vi "unflatten.vi"(8 "error in":errorcluster, 10 "flattened system":string) -> (0 "error out":errorcluster, 3 "test-system out":refnum<class "test-system.lvclass">)   [LabVIEW 2020, in "test-system.lvclass"]
uses:
  test-system.lvclass
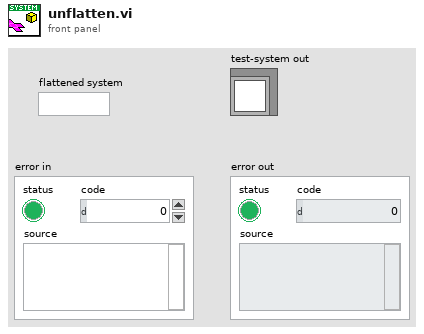
[diagram p1: front panel]
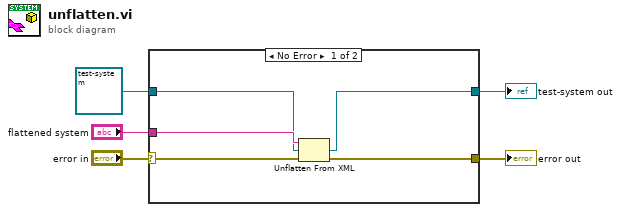
[diagram p0: block diagram]
diagram:
  n1 = case shown="No Error" "error in" {
    selector: "error in" -> [w7 w12]
    tunnel: [w6 w12] -> w4
    tunnel: [w8 w11] -> w2
    tunnel: refnum<class "test-system.lvclass"> refnum ("test-system in") -> [w9 w11]
    tunnel: "flattened system" -> [w10 _]
    frame No Error {
      n2 = Unflatten From XML(xml string=w10, type=w9, error in (no error)=w7) -> (value=w8:refnum<class "test-system.lvclass">, error out=w6:errorcluster)
    }
    frame Error {
    }
  }
  "error out" <- w4
  "test-system out" <- w2
